vi "CalculateTerminalVerticalCentre.vi"(8 "error in (no error)":errorcluster, 11 "ControlTerminal":refnum<vi>) -> (0 "error out":errorcluster, 2 "Terminal's vertical centre position":i32, 3 "ControlTerminal (dup)":refnum<vi>)   [LabVIEW 2017, in "ErrorStructureDrawer.lvlib"]
doc: "Calculates the vertical mid-point coordinate of the specified terminal - i.e. the point where a wire would enter or exit the terminal."
uses:
  ErrorStructureDrawer.lvlib
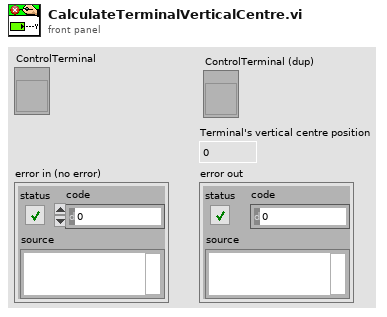
[diagram p1: front panel]
types:
  T1 = typedef "LVRectTypeDef.ctl" = cluster{"Left":i16, "Top":i16, "Right":i16, "Bottom":i16}
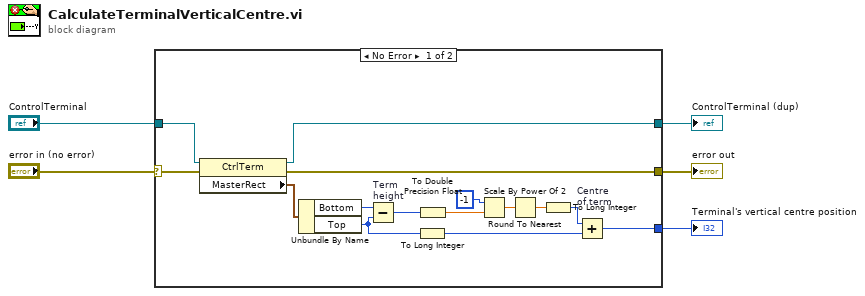
[diagram p0: block diagram]
diagram:
  n1 = case shown="No Error" "error in (no error)" {
    selector: "error in (no error)" -> [w8 w22]
    tunnel: [w20 w22] -> w5
    tunnel: "ControlTerminal" -> [w7 w21]
    tunnel: [w19 _] -> w3
    tunnel: [w6 w21] -> w1
    frame No Error {
      n2 = property class="CtrlTerm"(reference=w7, error in=w8) -> (reference out=w6:refnum<vi>, error out=w20:errorcluster, "MasterRect"=w9:T1)
      n3 = Unbundle By Name(w9) -> ("Bottom"=w10:i16, "Top"=w17:i16)
      n4 = Subtract "Term \nheight"(x=w10, y=w17) -> (x-y=w11:i16)
      n5 = To Long Integer(number=w17) -> (32bit integer=w18:i32)
      n6 = To Double Precision Float(number=w11) -> (double precision float=w12:dbl)
      n7 = Scale By Power Of 2(n=i16 -1, x=w12) -> (x*2^n=w14:dbl)
      n8 = Round To Nearest(number=w14) -> (nearest integer value=w15:dbl)
      n9 = To Long Integer(number=w15) -> (32bit integer=w16:i32)
      n10 = Add "Centre\nof term"(x=w16, y=w18) -> (x+y=w19:i32)
    }
    frame Error {
    }
  }
  "error out" <- w5
  "Terminal's vertical centre position" <- w3
  "ControlTerminal (dup)" <- w1
